vi "Attitude Control Write.vi"(8 "error in (no error)":errorcluster, 10 "pitch (x), roll (y), yaw (z)":T2, 11 "Attitude Control Handle In":T1) -> (0 "error out":errorcluster, 3 "Attitude Control Handle Out":T1)   [LabVIEW 2015, in "lv-attitudecontrol.lvlib"]
uses:
  lv-attitudecontrol.lvlib
  <vilib>/Utility/miscctls.llb/LV3DPointTypeDef.ctl
  Controls/AttitudeHandle.ctl
  <vilib>/picture/3D Picture Control/NI_3D Picture Control.lvlib
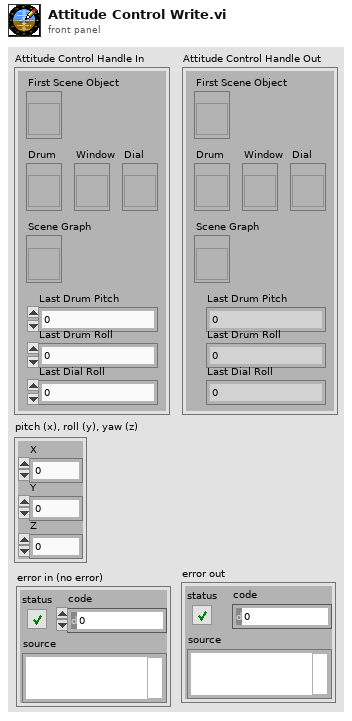
[diagram p1: front panel]
types:
  T1 = typedef "lv-attitudecontrol.lvlib/AttitudeHandle.ctl" = cluster{"First Scene Object":refnum<vi>, "Drum":refnum<vi>, "Window":refnum<vi>, "Dial":refnum<vi>, "Scene Graph":refnum<vi>, "Last Drum Pitch":dbl, "Last Drum Roll ":dbl, "Last Dial Roll":dbl}
  T2 = typedef "LV3DPointTypeDef.ctl" = cluster{"X":sgl, "Y":sgl, "Z":sgl}
  T3 = enum16{"None", "Spherical", "Flying", "Oriented"}
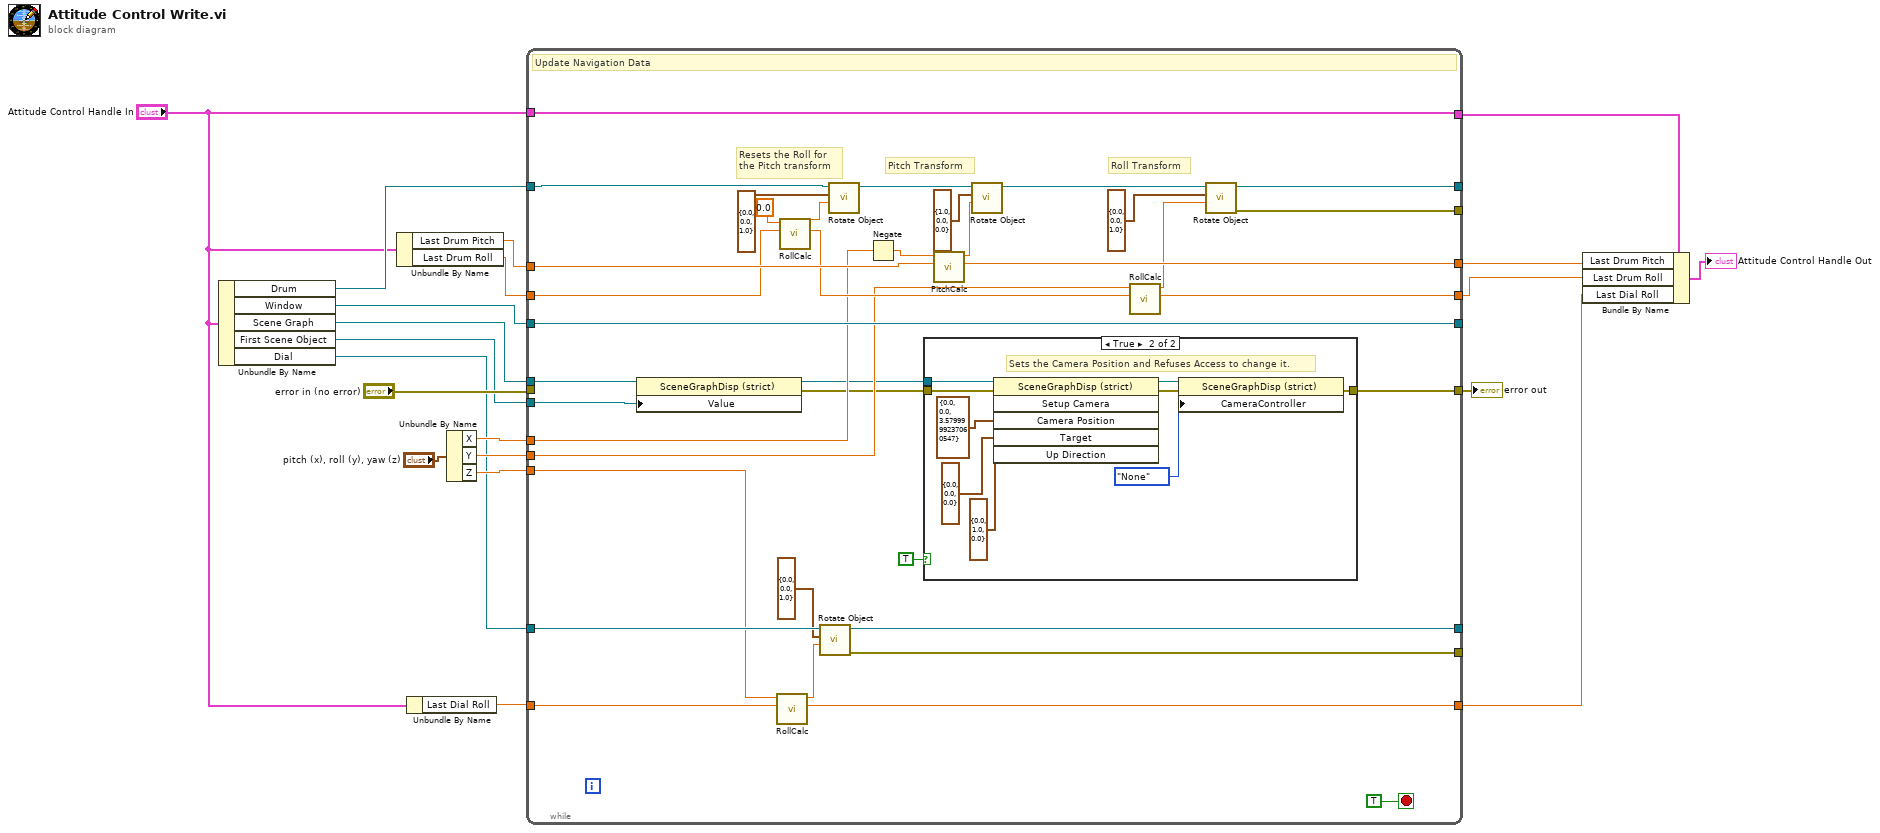
[diagram p0: block diagram]
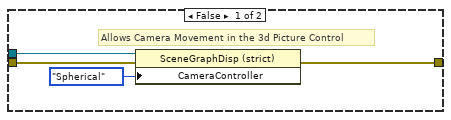
[diagram p2: hidden frame]
diagram:
  n1 = Unbundle By Name("Attitude Control Handle In") -> ("Drum"=w14:refnum<vi>, "Window"=w15:refnum<vi>, "Scene Graph"=w9:refnum<vi>, "First Scene Object"=w8:refnum<vi>, "Dial"=w7:refnum<vi>)
  n2 = Unbundle By Name("Attitude Control Handle In") -> ("Last Drum Pitch"=w12:dbl, "Last Drum Roll"=w11:dbl)
  n3 = Unbundle By Name("Attitude Control Handle In") -> ("Last Dial Roll"=w10:dbl)
  n4 = Unbundle By Name("pitch (x), roll (y), yaw (z)") -> ("X"=w18:sgl, "Y"=w19:sgl, "Z"=w20:sgl)
  n5 = while {
    tunnel: w15 -> [w56]
    tunnel: w14 -> [w24]
    tunnel: [w56] -> _
    tunnel: [w55] -> _
    tunnel: w7 -> [w48]
    tunnel: [w46] -> _
    tunnel: "error in (no error)" -> [_]
    tunnel: [w23] -> w13
    tunnel: w18 -> [w33]
    tunnel: w19 -> [w32]
    tunnel: w20 -> [w31]
    tunnel: w9 -> [w26]
    tunnel: w8 -> [w30]
    tunnel: "Attitude Control Handle In" -> [w25]
    tunnel: [w25] -> w4
    tunnel: w12 -> [w53]
    tunnel: [w52] -> w3
    tunnel: w11 -> [w50]
    tunnel: [w54] -> w2
    tunnel: w10 -> [w49]
    tunnel: [w47] -> w1
    tunnel: [w22] -> _
    tunnel: [w21] -> _
    stop <- TRUE stop-if-true
    # "Roll Transform"
    # "Resets the Roll for \nthe Pitch transform"
    # "Pitch Transform"
    # "Update Navigation Data"
    n6 = property on="Property Node" class="SceneGraphDisp (strict)"(reference=w26, "Value"=w30) -> (reference out=w28:refnum<vi>, error out=w29:errorcluster)  [unwired: 1 in]
    n7 = call "RollCalc.vi"("Previous Roll Value"=w49, "Roll Input"=w31) -> ("New Roll Value"=w47:dbl, "Adjustment to be Made"=w45:dbl)  [unwired: 8 in]
    n8 = call "RollCalc.vi"("Previous Roll Value"=w50, "Roll Input"=sgl 0.0 ("Angle")) -> ("New Roll Value"=w51:dbl, "Adjustment to be Made"=w40:dbl)  [unwired: 8 in]
    n9 = call <vilib>:"Rotate Object.vi"("Angle"=w45, "Axis"=cluster{"X":sgl, "Y":sgl, "Z":sgl} {"X"=0.0, "Y"=0.0, "Z"=1.0} ("Axis 2"), "Scene.Object In"=w48) -> ("error out"=w21:errorcluster, "Scene.Object Out"=w46:refnum<vi>)  [unwired: 7 in]
    n10 = call <vilib>:"Rotate Object.vi"("Angle"=w40, "Axis"=cluster{"X":sgl, "Y":sgl, "Z":sgl} {"X"=0.0, "Y"=0.0, "Z"=1.0} ("Axis 2"), "Scene.Object In"=w24) -> ("Scene.Object Out"=w41:refnum<vi>)  [unwired: 7 in, 1 out]
    n11 = Negate(x=w33) -> (-x=w34:sgl)
    n12 = case shown="True" TRUE {
      tunnel: [w59 w64] -> w23
      tunnel: w29 -> [w61 w66]
      tunnel: w28 -> [w58 w63]
      frame False {
        # "Allows Camera Movement in the 3d Picture Control"
        n13 = property on="Property Node" class="SceneGraphDisp (strict)"(reference=w58, error in=w61, "CameraController"=T3."Spherical" ("Camera Controller:Type")) -> (error out=w59:errorcluster)  [unwired: 1 out]
      }
      frame True {
        # "Sets the Camera Position and Refuses Access to change it."
        n14 = invoke on="Invoke Node" class="SceneGraphDisp (strict)" method="Setup Camera"(reference=w63, error in=w66, "Camera Position"=T2 {"X"=0.0, "Y"=0.0, "Z"=3.58}, "Target"=T2 {"X"=0.0, "Y"=0.0, "Z"=0.0}, "Up Direction"=T2 {"X"=0.0, "Y"=1.0, "Z"=0.0}) -> (reference out=w62:refnum<vi>, error out=w65:errorcluster)  [unwired: 1 in, 4 out]
        n15 = property on="Property Node" class="SceneGraphDisp (strict)"(reference=w62, error in=w65, "CameraController"=T3."None" ("Camera Controller:Type")) -> (error out=w64:errorcluster)  [unwired: 1 out]
      }
    }
    n16 = call "PitchCalc.vi"("Previous Pitch Value"=w53, "Pitch Control"=w34) -> ("New Pitch Value"=w52:dbl, "Adjustment to be made"=w42:dbl)  [unwired: 8 in]
    n17 = call <vilib>:"Rotate Object.vi"("Angle"=w42, "Axis"=cluster{"X":sgl, "Y":sgl, "Z":sgl} {"X"=1.0, "Y"=0.0, "Z"=0.0} ("Axis 2"), "Scene.Object In"=w41) -> ("Scene.Object Out"=w57:refnum<vi>)  [unwired: 7 in, 1 out]
    n18 = call "RollCalc.vi"("Previous Roll Value"=w51, "Roll Input"=w32) -> ("New Roll Value"=w54:dbl, "Adjustment to be Made"=w36:dbl)  [unwired: 8 in]
    n19 = call <vilib>:"Rotate Object.vi"("Angle"=w36, "Axis"=cluster{"X":sgl, "Y":sgl, "Z":sgl} {"X"=0.0, "Y"=0.0, "Z"=1.0} ("Axis 2"), "Scene.Object In"=w57) -> ("error out"=w22:errorcluster, "Scene.Object Out"=w55:refnum<vi>)  [unwired: 7 in]
  }
  "error out" <- w13
  n20 = Bundle By Name(cluster=w4, "Last Drum Pitch"=w3, "Last Drum Roll"=w2, "Last Dial Roll"=w1) -> (→"Attitude Control Handle Out":T1)
